vi "RT Driver VI.vi"(7 "Operation":T1, 11 "Device Reference in":T2 format="%.0x") -> (0 "Error Code":i32)   [LabVIEW 2025, in "Runtime Configuration Support Inline Async Example Engine.lvlib"]
uses:
  Runtime Configuration Support Inline Async Example Engine.lvlib
  <vilib>/NI VeriStand/Custom Device API/Custom Device Item Ref.ctl
  <vilib>/NI VeriStand/Custom Device API/Hardware Interface Driver VI Operation.ctl
  Shared/Compiled.Settings.ctl
  <vilib>/NI/NIVS Inline Async API/_VS Inline Async API/VS Inline Async API/VS Inline Async API.lvclass
  Shared/Parameter.ctl
  Shared/AsyncRequest.ctl
  Shared/ReConfigured.Settings.ctl
  <vilib>/NI VeriStand/Custom Device API/Block Data Reference.ctl
  <vilib>/NI VeriStand/Custom Device API/Data Reference.ctl
  <vilib>/NI/NIVS Inline Async API/_VS Inline Async API/VS Inline Async API/VS Inline Async API.lvclass/VS Inline Async API.ctl
  <vilib>/NI/NIVS Inline Async API/_Data Access Engine/Data Access Engine/Data Access Engine.lvclass/Data Access Engine.ctl
  <vilib>/NI/NIVS Inline Async API/_Data Access Engine/Access Type Classes/Write/Write.lvclass/Write.ctl
  <vilib>/NI/NIVS Inline Async API/_Data Access Engine/Access Type Classes/ReadWrite/ReadWrite.lvclass/ReadWrite.ctl
  <vilib>/NI/NIVS Inline Async API/_Data Access Engine/Access Type Classes/Read/Read.lvclass/Read.ctl
  <vilib>/NI/NIVS Inline Async API/_Data Access Engine/Data Access Engine/Methods/Data.Engine.Read Data from HW.vi
  <vilib>/NI/NIVS Inline Async API/_VS Inline Async API/Error Handling Process/SubVIs/Error.GetError.vi
  <vilib>/NI/NIVS Inline Async API/_Data Access Engine/Data Access Engine/Methods/Data.Engine.Write Data to HW.vi
  <vilib>/NI/NIVS Inline Async API/_Data Access Engine/Access Type Classes/ReadWrite/ReadWrite.EngineData.vi
  <vilib>/NI/NIVS Inline Async API/_Data Access Engine/Access Type Classes/Write/Write.EngineData.vi
  <vilib>/NI/NIVS Inline Async API/_Data Access Engine/Access Type Classes/Read/Read.EngineData.vi
  <vilib>/NI VeriStand/Custom Device API/NI VeriStand - Get Channel Value by Data Reference.vi
  <vilib>/NI VeriStand/Custom Device API/NI VeriStand - Set Channel Value by Data Reference.vi
  <vilib>/NI VeriStand/Custom Device API/NI VeriStand - Set Channel Values by Block Data Reference.vi
  <vilib>/NI VeriStand/Custom Device API/NI VeriStand - Get Channel Values by Block Data Reference.vi
  Runtime Configuration Support Inline Async Example.Async.vi
  Command Loop.vi
  Shared/Constants.vi
  <vilib>/NI VeriStand/Custom Device API/Get Item Property (Variant).vi
  <vilib>/NI VeriStand/Custom Device API/Global Data Refs.vi
  <vilib>/NI VeriStand/Custom Device Tools/Custom Device Utility Library/Custom Device Utility Library.lvlib
  Shared/Runtime Configuration Support Inline Async Example Shared.lvlib
  <vilib>/NI VeriStand/Custom Device API/Custom Device API.lvlib
  <vilib>/NI/NIVS Inline Async API/_Data Access Engine/Data Access Engine/Data Access Engine.lvclass
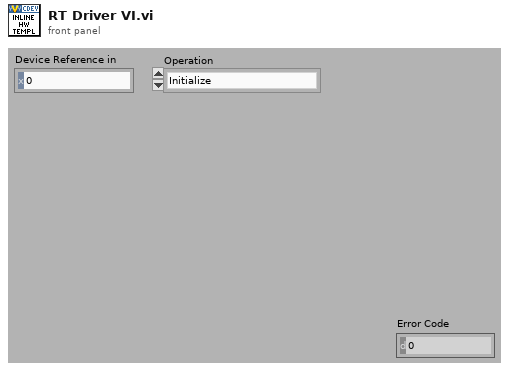
[diagram p1: front panel]
types:
  T1 = typedef "Custom Device API.lvlib/Hardware Interface Driver VI Operation.ctl" = enum16{"Initialize", "Start", "Read Data from HW", "Write Data to HW", "Close"}
  T2 = typedef "Custom Device API.lvlib/Custom Device Item Ref.ctl" = u64
  T3 = typedef "Runtime Configuration Support Inline Async Example Engine.lvlib/Parameter.ctl" = cluster{"Compiled.Settings":T4, "Async Request Ref":refnum<queue>}
  T4 = typedef "Runtime Configuration Support Inline Async Example Shared.lvlib/Compiled.Settings.ctl" = cluster{"Name":string, "Async Init Timeout":u16, "Inport SignalIDs":i32[], "Outport SignalIDs":i32[], "Inport Values":dbl[], "Outport Values":dbl[], "Dynamic Config Status":bool, "Device Error":errorcluster}
  T5 = typedef "Runtime Configuration Support Inline Async Example Shared.lvlib/ReConfigured.Settings.ctl" = cluster{"Compiled.Settings":T4, "Compiled Inline Async Settings":cluster{"Read":cluster{"Refs":T6[], "Values":dbl[]}[], "Write":cluster{"Refs":T6[], "Values":dbl[]}[], "ReadWrite":cluster{"Refs":T7[], "Values":dbl[], "Reset Values":dbl[]}[], "LUT":variant}, "Response Ref":refnum<queue>}
  T6 = typedef "Custom Device API.lvlib/Block Data Reference.ctl" = cluster{"Data Reference":T7, "Offset":u64, "Length":u64}
  T7 = typedef "Custom Device API.lvlib/Data Reference.ctl" = i32
  T8 = cluster{"Async":refnum<class "VS Inline Async API.lvclass">, "Parameter":T3, "ReConfigured.Settings":T5}
  T9 = cluster{"ReConfigured.Settings Ref":refnum<queue>}
  T10 = typedef "Runtime Configuration Support Inline Async Example Engine.lvlib/AsyncRequest.ctl" = cluster{"Compiled.Settings":T4, "Data Access":variant, "Async Response Ref":refnum<queue>}
  T11 = cluster{"Dynamic Config Status":bool, "Error":errorcluster}
  T12 = cluster{"Read":cluster{"Refs":T6[], "Values":dbl[]}[], "Write":cluster{"Refs":T6[], "Values":dbl[]}[], "ReadWrite":cluster{"Refs":T7[], "Values":dbl[], "Reset Values":dbl[]}[], "LUT":variant}
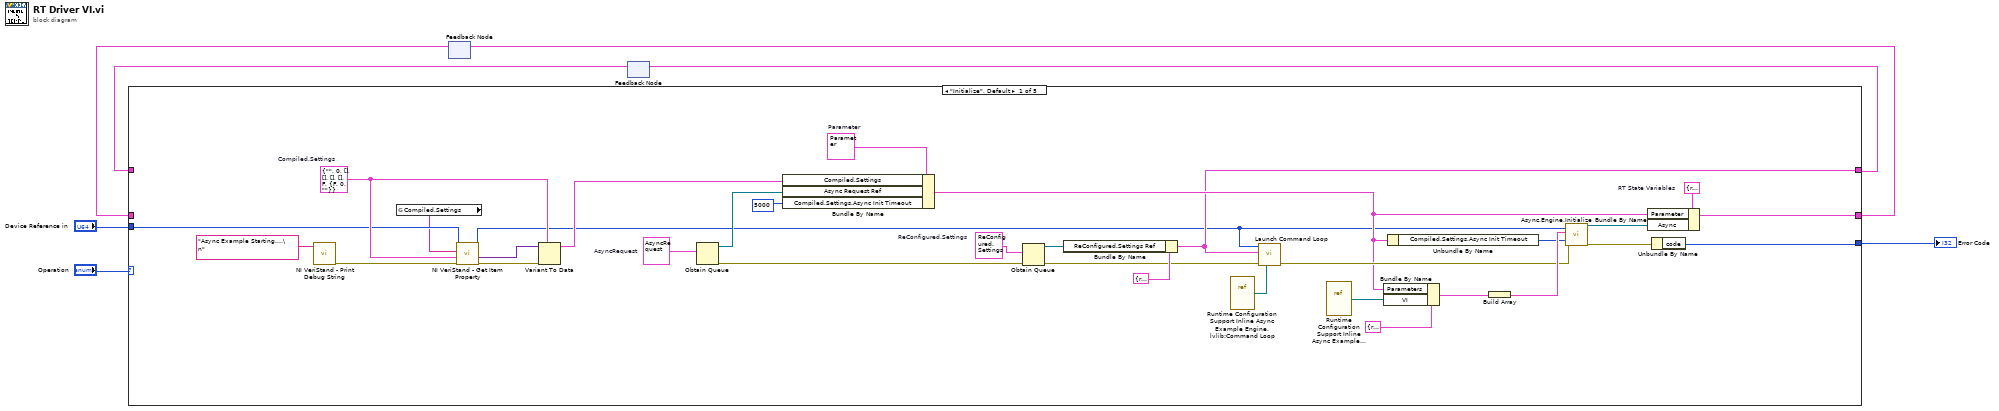
[diagram p0: block diagram]
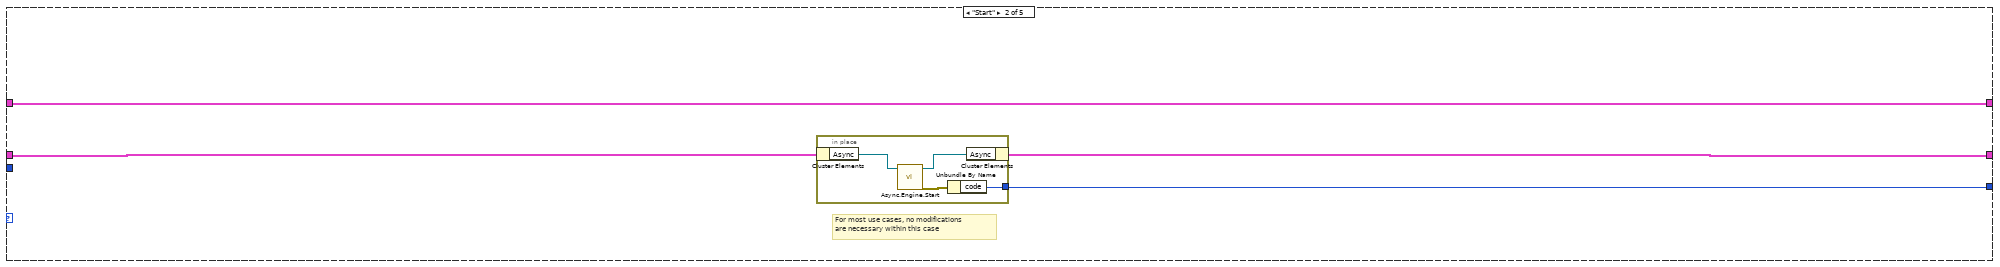
[diagram p2: hidden frame]
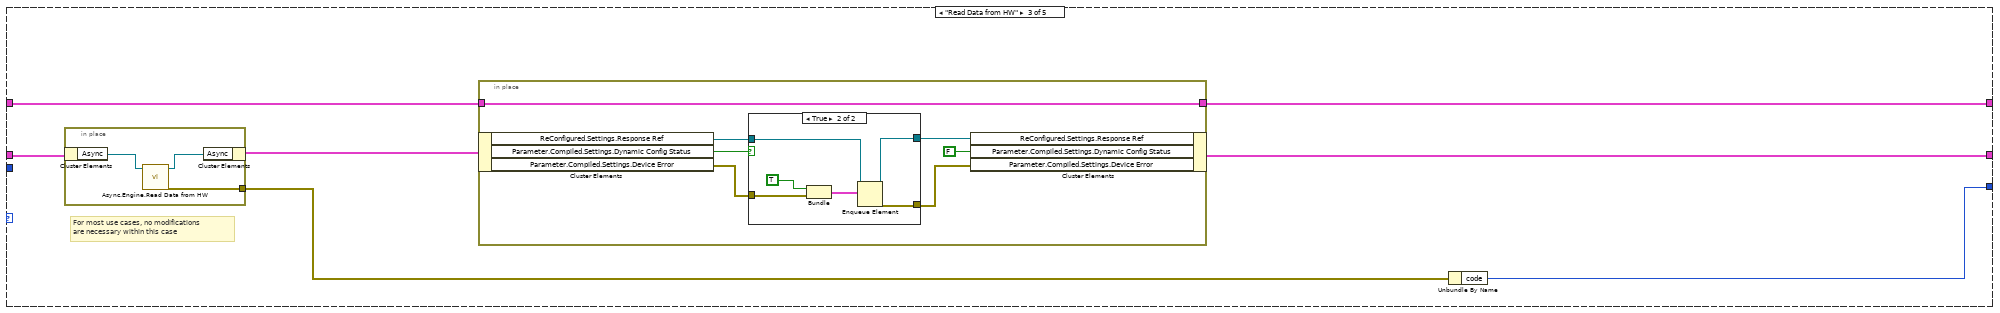
[diagram p3: hidden frame]
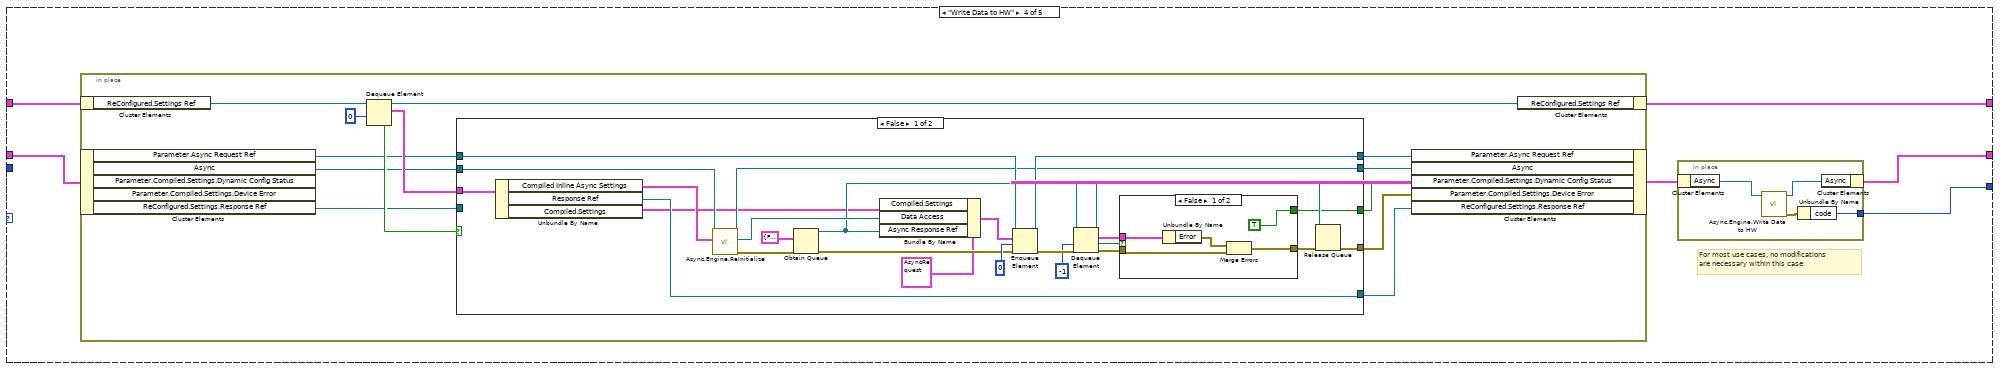
[diagram p5: hidden frame]
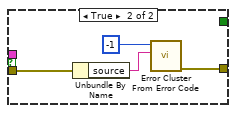
[diagram p6: hidden frame]
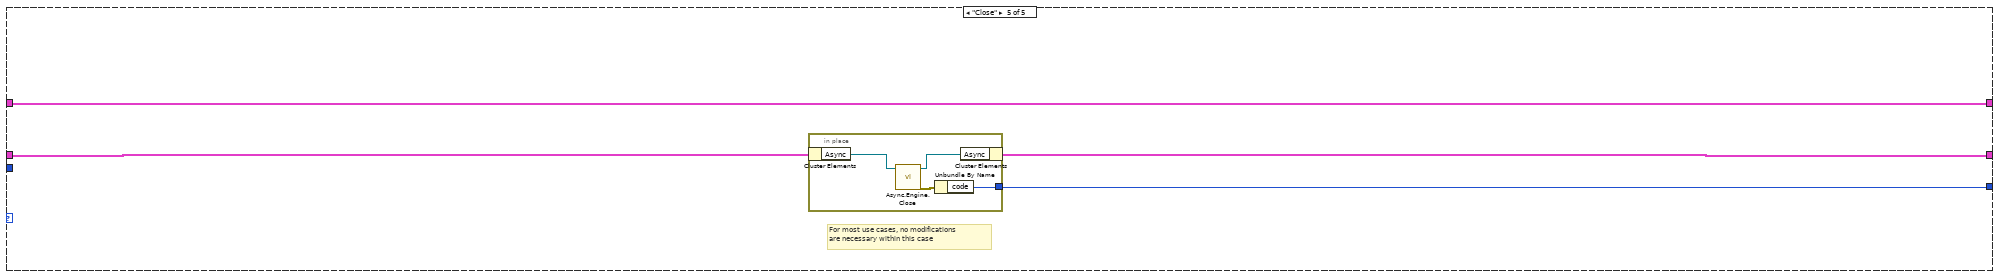
[diagram p8: hidden frame]
diagram:
  n1 = feedback #1() -> (w5:T8)  [unwired: 1 out]
  n2 = feedback #2() -> (w1:T9)  [unwired: 1 in]
  n3 = case shown="\"Initialize\", Default" "Operation" {
    tunnel: [w37 w42 w52 w77 w135] -> w6
    tunnel: w5 -> [_ w43 w54 w73 w136]
    tunnel: "Device Reference in" -> [w24 _ _ _ _]
    tunnel: [w39 w41 w50 w78 w134] -> w3
    tunnel: [w15 w40 w49 w75 w133] -> w2
    tunnel: w1 -> [_ w40 w48 w76 w133]
    frame "Initialize", Default {
      w12 = T5 {"Compiled.Settings"={"Name"="", "Async Init Timeout"=0, "Inport SignalIDs"=[], "Outport SignalIDs"=[], "Inport Values"=[], "Outport Values"=[], "Dynamic Config Status"=FALSE, "Device Error"={"status"=FALSE, "code"=0, "source"=""}}, "Compiled Inline Async Settings"={"Read"=[], "Write"=[], "ReadWrite"=[], "LUT"=variant}, "Response Ref"=refnum}  # ReConfigured.Settings
      w19 = T10 {"Compiled.Settings"={"Name"="", "Async Init Timeout"=0, "Inport SignalIDs"=[], "Outport SignalIDs"=[], "Inport Values"=[], "Outport Values"=[], "Dynamic Config Status"=FALSE, "Device Error"={"status"=FALSE, "code"=0, "source"=""}}, "Data Access"=variant(u16 0), "Async Response Ref"=refnum}  # AsyncRequest
      w16 = T3 {"Compiled.Settings"={"Name"="", "Async Init Timeout"=0, "Inport SignalIDs"=[], "Outport SignalIDs"=[], "Inport Values"=[], "Outport Values"=[], "Dynamic Config Status"=FALSE, "Device Error"={"status"=FALSE, "code"=0, "source"=""}}, "Async Request Ref"=refnum}  # Parameter
      w34 = T8 {"Async"=refnum, "Parameter"={"Compiled.Settings"={"Name"="", "Async Init Timeout"=0, "Inport SignalIDs"=[], "Outport SignalIDs"=[], "Inport Values"=[], "Outport Values"=[], "Dynamic Config Status"=FALSE, "Device Error"={"status"=FALSE, "code"=0, "source"=""}}, "Async Request Ref"=refnum}, "ReConfigured.Settings"={"Compiled.Settings"={"Name"="", "Async Init Timeout"=0, "Inport SignalIDs"=[], "Outport SignalIDs"=[], "Inport Values"=[], "Outport Values"=[], "Dynamic Config Status"=FALSE, "Device Error"={"status"=FALSE, "code"=0, "source"=""}}, "Compiled Inline Async Settings"={"Read"=[], "Write"=[], "ReadWrite"=[], "LUT"=variant}, "Response Ref"=refnum}}  # RT State Variables
      w25 = T4 {"Name"="", "Async Init Timeout"=0, "Inport SignalIDs"=[], "Outport SignalIDs"=[], "Inport Values"=[], "Outport Values"=[], "Dynamic Config Status"=FALSE, "Device Error"={"status"=FALSE, "code"=0, "source"=""}}  # Compiled.Settings
      n4 = call <vilib>:"NI VeriStand - Print Debug String.vi"("Message"="Async Example Starting....\n") -> ("error out"=w30:errorcluster)  [unwired: 10 in]
      n5 = global read "Constants.vi" "Compiled.Settings"() -> (w22:string)
      n6 = call-poly <vilib>:"NI VeriStand - Get Item Property.vi"("error in (no error)"=w30, "Default Value"=w25, "Property Name"=w22, "Item Ref in"=w24) -> ("error out"=w21:errorcluster, "Value"=w23:variant, "Item Ref out"=w9:T2)  [unwired: 4 in, 1 out]
      n7 = Variant To Data(error in=w21, type=w25, Variant=w23) -> (data=w20:T4)  [unwired: 1 out]
      n8 = Obtain Queue(element data type=w19) -> (queue out=w18:refnum<queue>, error out=w8:errorcluster)  [unwired: 4 in, 1 out]
      n9 = Bundle By Name(cluster=w16, "Compiled.Settings"=w20, "Async Request Ref"=w18, "Compiled.Settings.Async Init Timeout"=u16 5000) -> (w17:T3)
      n10 = Obtain Queue(element data type=w12, error in (no error)=w8) -> (queue out=w11:refnum<queue>, error out=w13:errorcluster)  [unwired: 3 in, 1 out]
      n11 = Bundle By Name(cluster=T9 {"ReConfigured.Settings Ref"=refnum} ("Queue Refs"), "ReConfigured.Settings Ref"=w11) -> (w15:T9)
      n12 = vi-ref "Runtime Configuration Support Inline Async Example Engine.lvlib:Command Loop.vi"() -> (w27:refnum<vi>)
      n13 = call "Launch Command Loop.vi"("VI Refnum"=w27, "error in"=w13, "Queue Refs"=w15, "Device Reference in"=w9) -> ("error out"=w26:errorcluster)  [unwired: 7 in]
      n14 = vi-ref "Runtime Configuration Support Inline Async Example Engine.lvlib:Runtime Configuration Support Inline Async Example.Async.vi"() -> (w31:refnum<vi>)
      n15 = Bundle By Name(cluster=cluster{"VI":refnum<vi>, "Parameters":variant} {"VI"=refnum, "Parameters"=variant} ("Process"), "Parameters"=w17, "VI"=w31) -> (w35:cluster{"VI":refnum<vi>, "Parameters":variant})
      n16 = Unbundle By Name(w17) -> ("Compiled.Settings.Async Init Timeout"=w29:u16)
      n17 = Build Array(w35) -> (w33:cluster{"VI":refnum<vi>, "Parameters":variant}[])
      n18 = call <vilib>:"Async.Engine.Initialize.vi"("Timeout (ms) (5000)"=w29, "error in (no error)"=w26, "Processes"=w33, "Custom Device Ref"=w9) -> ("error out"=w28:errorcluster, "Async"=w38:refnum<class "VS Inline Async API.lvclass">)  [unwired: 6 in]
      n19 = Bundle By Name(cluster=w34, "Parameter"=w17, "Async"=w38) -> (w37:T8)
      n20 = Unbundle By Name(w28) -> ("code"=w39:i32)
    }
    frame "Start" {
      # "For most use cases, no modifications \nare necessary within this case"
      n21 = in-place {
        in-place-border: [w44] -> w41
        n22 = in-place-cluster #3(w43) -> ("Async"=w47:refnum<class "VS Inline Async API.lvclass">)
        n23 = call <vilib>:"Async.Engine.Start.vi"("VS Inline Async API in"=w47) -> ("error out"=w45:errorcluster, "VS Inline Async API out"=w46:refnum<class "VS Inline Async API.lvclass">)  [unwired: 9 in]
        n24 = Unbundle By Name(w45) -> ("code"=w44:i32)
        n25 = in-place-cluster #3("Async"=w46) -> (w42:T8)
      }
    }
    frame "Read Data from HW" {
      # "For most use cases, no modifications \nare necessary within this case"
      n26 = in-place {
        in-place-border: [w70] -> w51
        n27 = in-place-cluster #4(w54) -> ("Async"=w72:refnum<class "VS Inline Async API.lvclass">)
        n28 = call <vilib>:"Async.Engine.Read Data from HW.vi"("Async in"=w72) -> ("error out"=w70:errorcluster, "Async out"=w71:refnum<class "VS Inline Async API.lvclass">)  [unwired: 9 in]
        n29 = in-place-cluster #4("Async"=w71) -> (w53:T8)
      }
      n30 = in-place {
        in-place-border: [w55] -> w49
        in-place-border: w48 -> [w55]
        n31 = in-place-cluster #5(w53) -> ("ReConfigured.Settings.Response Ref"=w57:refnum<queue>, "Parameter.Compiled.Settings.Dynamic Config Status"=w61:bool, "Parameter.Compiled.Settings.Device Error"=w60:errorcluster)
        n32 = case shown="True" w61 {
          tunnel: [w62 w69] -> w56
          tunnel: w60 -> [w63 w67]
          tunnel: [w63 w64] -> w59
          tunnel: w57 -> [w62 w65]
          frame False {
          }
          frame True {
            n33 = Bundle(TRUE, "Device Error"=w67) -> (w66:cluster{bool, "Device Error":errorcluster})  [unwired: 1 in]
            n34 = Enqueue Element(queue=w65, element=w66) -> (queue out=w69:refnum<queue>, error out=w64:errorcluster)  [unwired: 2 in, 1 out]
          }
        }
        n35 = in-place-cluster #5("ReConfigured.Settings.Response Ref"=w56, "Parameter.Compiled.Settings.Dynamic Config Status"=FALSE ("Compiled.Settings.Compiled Info.Dynamic Config Status"), "Parameter.Compiled.Settings.Device Error"=w59) -> (w52:T8)
      }
      n36 = Unbundle By Name(w51) -> ("code"=w50:i32)
    }
    frame "Write Data to HW" {
      # "For most use cases, no modifications \nare necessary within this case"
      n37 = in-place {
        n38 = in-place-cluster #6(w76) -> ("ReConfigured.Settings Ref"=w86:refnum<queue>)
        n39 = in-place-cluster #7(w73) -> ("Parameter.Async Request Ref"=w88:refnum<queue>, "Async"=w84:refnum<class "VS Inline Async API.lvclass">, "ReConfigured.Settings.Response Ref"=w80:refnum<queue>)  [unwired: 2 out]
        n40 = Dequeue Element(queue=w86, timeout in ms (-1)=0) -> (queue out=w85:refnum<queue>, element=w89:T5, timed out?=w90:bool)  [unwired: 1 in, 1 out]
        n41 = case shown="False" w90 {
          tunnel: w89 -> [w113 _]
          tunnel: w88 -> [w114 w128]
          tunnel: [w115 w128] -> w87
          tunnel: w84 -> [w110 w127]
          tunnel: [w109 w127] -> w83
          tunnel: [w98 _] -> w81
          tunnel: [w96 _] -> w82
          tunnel: w80 -> [_ w126]
          tunnel: [w93 w126] -> w79
          frame False {
            n42 = Unbundle By Name(w113) -> ("Compiled Inline Async Settings"=w108:T12, "Response Ref"=w93:refnum<queue>, "Compiled.Settings"=w92:T4)
            n43 = call <vilib>:"Async.Engine.ReInitialize.vi"("Compiled Inline Async"=w108, "Async in"=w110) -> ("error out"=w106:errorcluster, "Data Access Engine"=w107:refnum<class "Data Access Engine.lvclass">, "Async out"=w109:refnum<class "VS Inline Async API.lvclass">)  [unwired: 7 in]
            n44 = Obtain Queue(element data type=T11 {"Dynamic Config Status"=FALSE, "Error"={"status"=FALSE, "code"=0, "source"=""}}, error in (no error)=w106) -> (queue out=w95:refnum<queue>, error out=w105:errorcluster)  [unwired: 3 in, 1 out]
            n45 = Bundle By Name(cluster=T10 {"Compiled.Settings"={"Name"="", "Async Init Timeout"=0, "Inport SignalIDs"=[], "Outport SignalIDs"=[], "Inport Values"=[], "Outport Values"=[], "Dynamic Config Status"=FALSE, "Device Error"={"status"=FALSE, "code"=0, "source"=""}}, "Data Access"=variant, "Async Response Ref"=refnum} ("AsyncRequest"), "Compiled.Settings"=w92, "Data Access"=w107, "Async Response Ref"=w95) -> (w111:T10)
            n46 = Enqueue Element(queue=w114, element=w111, timeout in ms (-1)=0, error in (no error)=w105) -> (queue out=w115:refnum<queue>, error out=w104:errorcluster)  [unwired: 1 out]
            n47 = Dequeue Element(queue=w95, timeout in ms (-1)=-1, error in (no error)=w104) -> (queue out=w99:refnum<queue>, element=w97:T11, timed out?=w102:bool, error out=w101:errorcluster)
            n48 = case shown="False" w102 {
              tunnel: w101 -> [w118 w124]
              tunnel: [w117 w122] -> w100
              tunnel: w97 -> [w120 _]
              tunnel: [TRUE ("Dynamic Config Status") _] -> w96
              frame False {
                n49 = Unbundle By Name(w120) -> ("Error"=w119:errorcluster)
                n50 = Merge Errors(w119, w118) -> (w117:errorcluster)
              }
              frame True {
                n51 = Unbundle By Name(w124) -> ("source"=w123:string)
                n52 = call <vilib>:"Error Cluster From Error Code.vi"("error message (\"\")"=w123, "error code (0)"=-1) -> ("error out"=w122:errorcluster)  [unwired: 7 in]
              }
            }
            n53 = Release Queue(queue=w99, error in (no error)=w100) -> (error out=w98:errorcluster)  [unwired: 1 in, 2 out]
          }
          frame True {
          }
        }
        n54 = in-place-cluster #7("Parameter.Async Request Ref"=w87, "Async"=w83, "Parameter.Compiled.Settings.Dynamic Config Status"=w82, "Parameter.Compiled.Settings.Device Error"=w81, "ReConfigured.Settings.Response Ref"=w79) -> (w74:T8)
        n55 = in-place-cluster #6("ReConfigured.Settings Ref"=w85) -> (w75:T9)
      }
      n56 = in-place {
        in-place-border: [w132] -> w78
        n57 = in-place-cluster #8(w74) -> ("Async"=w130:refnum<class "VS Inline Async API.lvclass">)
        n58 = call <vilib>:"Async.Engine.Write Data to HW.vi"("VS Inline Async API in"=w130) -> ("error out"=w131:errorcluster, "VS Inline Async API out"=w129:refnum<class "VS Inline Async API.lvclass">)  [unwired: 9 in]
        n59 = Unbundle By Name(w131) -> ("code"=w132:i32)
        n60 = in-place-cluster #8("Async"=w129) -> (w77:T8)
      }
    }
    frame "Close" {
      # "For most use cases, no modifications \nare necessary within this case"
      n61 = in-place {
        in-place-border: [w138] -> w134
        n62 = in-place-cluster #9(w136) -> ("Async"=w140:refnum<class "VS Inline Async API.lvclass">)
        n63 = call <vilib>:"Async.Engine.Close.vi"("Async in"=w140) -> ("error out"=w137:errorcluster, "Async out"=w139:refnum<class "VS Inline Async API.lvclass">)  [unwired: 9 in]
        n64 = Unbundle By Name(w137) -> ("code"=w138:i32)
        n65 = in-place-cluster #9("Async"=w139) -> (w135:T8)
      }
    }
  }
  "Error Code" <- w3
  n66 = feedback-in #1(w6) -> ()
  n67 = feedback-in #2(w2) -> ()
